vi "Send Packet by UART.vi"(2 "기타 설정":T1={"필터종류"=0, "속도 ID"=1, "출력 주기"=0, "필터 세부 정보"=0, "송수신 ID"=[]} {"출력 주기" items=["200Hz", "10Hz", "20Hz", "50Hz", "100Hz", "200Hz", "333Hz", "500Hz", "1000Hz"]; "속도 ID" items=["1 Mbps"=1, "500Kbps"=2, "250Kbps"=3, "125Kbps"=4, "100Kbps"=5]; "필터종류" items=["None", "LowPass Filter"]}, 3 "Command":u16(ring) items=["제품명 읽기", "S/N 읽기", "Firmware Version 읽기", "제품 ID 설정", "제품 ID 읽기", "통신 속도 설정", "통신 속도 읽기", "필터 종류 설정", "필터 종류 읽기", "F/T 현재값 출력", "F/T 연속 출력", "F/T 출력 멈춤", "Reserved", "Reserved", "출력 주기 설정", "출력 주기 읽기", "Bias 설정", "Overload log 읽기"]) -> (0 "탭 컨트롤":enum32{"통신 속도", "송수신 ID", "필터", "출력주기"}(tab), 1 "Packet":u8[](array[numeric]))   [LabVIEW 2011]
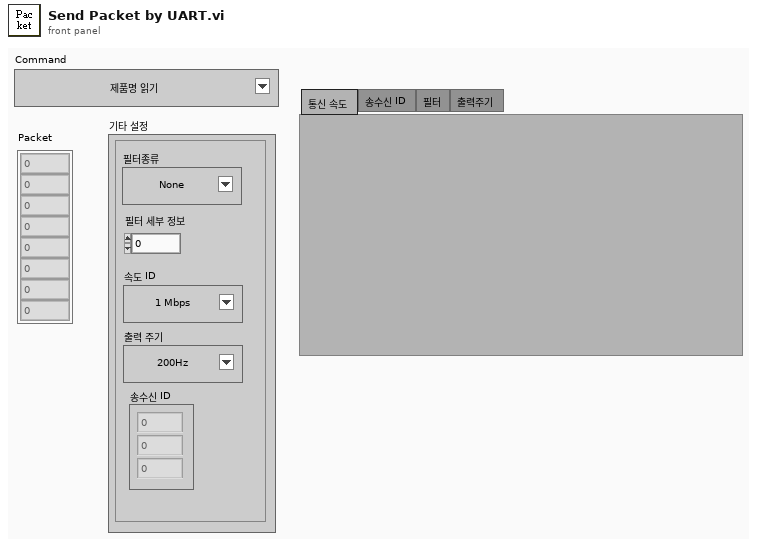
[diagram p1: front panel]
types:
  T1 = cluster{"필터종류":u16, "속도 ID":u16, "출력 주기":u16, "필터 세부 정보":u8, "송수신 ID":u8[]}
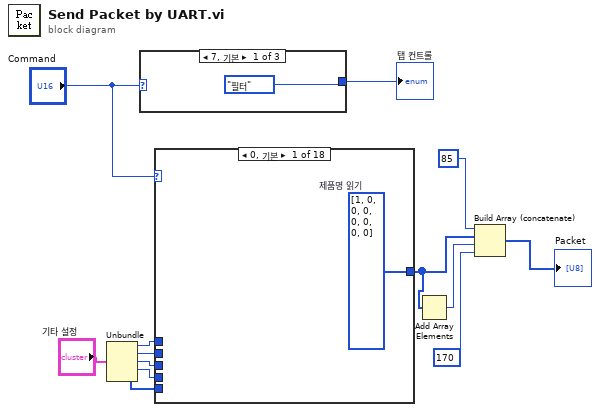
[diagram p0: block diagram]
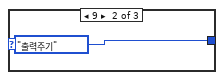
[diagram p2: hidden frame]
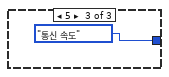
[diagram p3: hidden frame]
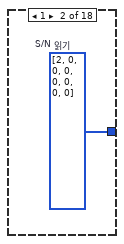
[diagram p4: hidden frame]
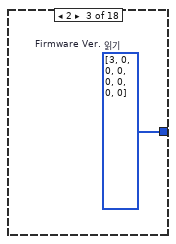
[diagram p5: hidden frame]
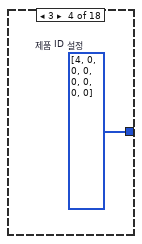
[diagram p6: hidden frame]
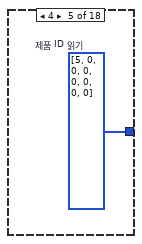
[diagram p7: hidden frame]
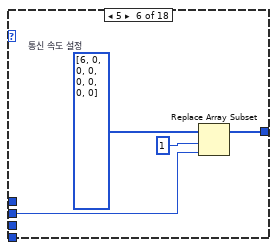
[diagram p8: hidden frame]
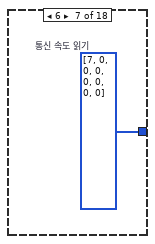
[diagram p9: hidden frame]
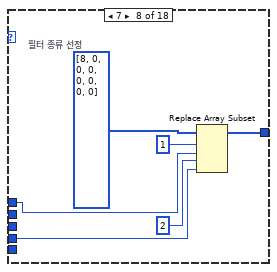
[diagram p10: hidden frame]
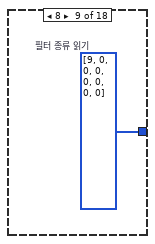
[diagram p11: hidden frame]
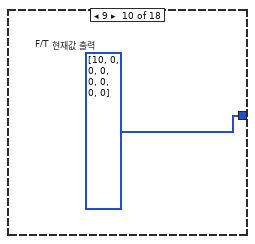
[diagram p12: hidden frame]
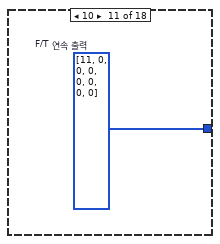
[diagram p13: hidden frame]
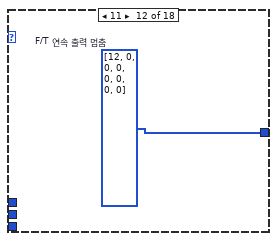
[diagram p14: hidden frame]
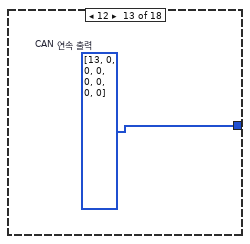
[diagram p15: hidden frame]
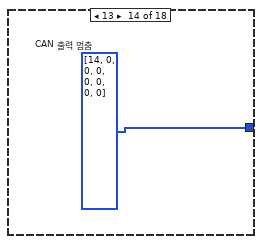
[diagram p16: hidden frame]
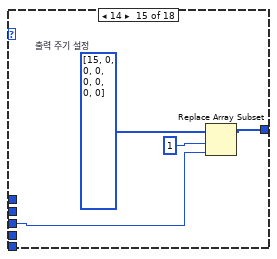
[diagram p17: hidden frame]
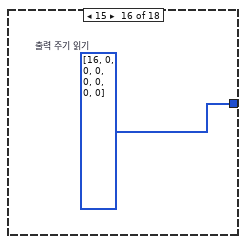
[diagram p18: hidden frame]
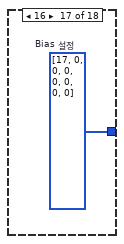
[diagram p19: hidden frame]
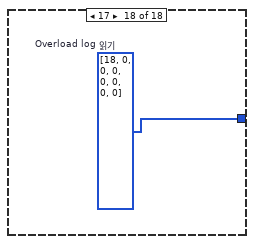
[diagram p20: hidden frame]
diagram:
  n1 = Unbundle("기타 설정") -> ("필터종류"=w11:u16, "속도 ID"=w12:u16, "출력 주기"=w9:u16, "필터 세부 정보"=w10:u8, "송수신 ID"=w6:u8[])
  n2 = case shown="7, 기본" "Command" {
    tunnel: [enum32{"통신 속도", "송수신 ID", "필터", "출력주기"}."필터" ("탭 컨트롤") enum32{"통신 속도", "송수신 ID", "필터", "출력주기"}."출력주기" ("탭 컨트롤") enum32{"통신 속도", "송수신 ID", "필터", "출력주기"}."통신 속도" ("탭 컨트롤")] -> w7
    frame 7, Default {
    }
    frame 9 {
    }
    frame 5 {
    }
  }
  "탭 컨트롤" <- w7
  n3 = case shown="0, 기본" "Command" {
    tunnel: [w17 w18 w19 w20 w21 w23 w26 w29 w33 w34 w35 w36 w37 w38 w40 w43 w44 w45] -> w3
    tunnel: w12 -> [_ _ _ _ _ w22 _ _ _ _ _ _ _ _ _ _ _ _]
    tunnel: w11 -> [_ _ _ _ _ _ _ w28 _ _ _ _ _ _ _ _ _ _]
    tunnel: w10 -> [_ _ _ _ _ _ _ w27 _ _ _ _ _ _ _ _ _ _]
    tunnel: w9 -> [_ _ _ _ _ _ _ _ _ _ _ _ _ _ w39 _ _ _]
    tunnel: w6 -> [_ _ _ _ _ _ _ _ _ _ _ _ _ _ _ _ _ _]
    frame 0, Default {
      w17 = u8[] [1, 0, 0, 0, 0, 0, 0, 0]  # 제품명 읽기
    }
    frame 1 {
      w18 = u8[] [2, 0, 0, 0, 0, 0, 0, 0]  # S/N 읽기
    }
    frame 2 {
      w19 = u8[] [3, 0, 0, 0, 0, 0, 0, 0]  # Firmware Ver. 읽기
    }
    frame 3 {
      w20 = u8[] [4, 0, 0, 0, 0, 0, 0, 0]  # 제품 ID 설정
    }
    frame 4 {
      w21 = u8[] [5, 0, 0, 0, 0, 0, 0, 0]  # 제품 ID 읽기
    }
    frame 5 {
      w24 = u8[] [6, 0, 0, 0, 0, 0, 0, 0]  # 통신 속도 설정
      n4 = Replace Array Subset(array=w24, new element=w22, index=1 ("인덱스")) -> (w23:u8[])
    }
    frame 6 {
      w26 = u8[] [7, 0, 0, 0, 0, 0, 0, 0]  # 통신 속도 읽기
    }
    frame 7 {
      w31 = u8[] [8, 0, 0, 0, 0, 0, 0, 0]  # 필터 종류 선정
      n5 = Replace Array Subset(array=w31, new element #1=w28, index #1=1 ("인덱스"), new element #2=w27, index #2=2 ("인덱스")) -> (w29:u8[])
    }
    frame 8 {
      w33 = u8[] [9, 0, 0, 0, 0, 0, 0, 0]  # 필터 종류 읽기
    }
    frame 9 {
      w34 = u8[] [10, 0, 0, 0, 0, 0, 0, 0]  # F/T 현재값 출력
    }
    frame 10 {
      w35 = u8[] [11, 0, 0, 0, 0, 0, 0, 0]  # F/T 연속 출력
    }
    frame 11 {
      w36 = u8[] [12, 0, 0, 0, 0, 0, 0, 0]  # F/T 연속 출력 멈춤
    }
    frame 12 {
      w37 = u8[] [13, 0, 0, 0, 0, 0, 0, 0]  # CAN 연속 출력
    }
    frame 13 {
      w38 = u8[] [14, 0, 0, 0, 0, 0, 0, 0]  # CAN 출력 멈춤
    }
    frame 14 {
      w42 = u8[] [15, 0, 0, 0, 0, 0, 0, 0]  # 출력 주기 설정
      n6 = Replace Array Subset(array=w42, new element=w39, index=1 ("인덱스")) -> (w40:u8[])
    }
    frame 15 {
      w43 = u8[] [16, 0, 0, 0, 0, 0, 0, 0]  # 출력 주기 읽기
    }
    frame 16 {
      w44 = u8[] [17, 0, 0, 0, 0, 0, 0, 0]  # Bias 설정
    }
    frame 17 {
      w45 = u8[] [18, 0, 0, 0, 0, 0, 0, 0]  # Overload log 읽기
    }
  }
  n7 = Add Array Elements(numeric array=w3) -> (sum=w2:u8)
  n8 = Build Array (concatenate)(85, w3, w2, 170) -> (→"Packet":i32[])
